vi "BUZZER_CONTROL.vi"() -> ()   [LabVIEW 2015]
panel:
  in  "Buzzer Control":bool
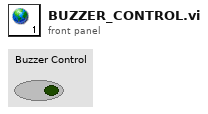
[diagram p1: front panel]
diagram:
